vi "SwitchingFieldDistribution.vi"(1 "B":dbl[](array[numeric]), 2 "H":dbl[](array[numeric])) -> (0 "SFD":dbl)   [LabVIEW 2019]
panel:
  out "error out":errorcluster
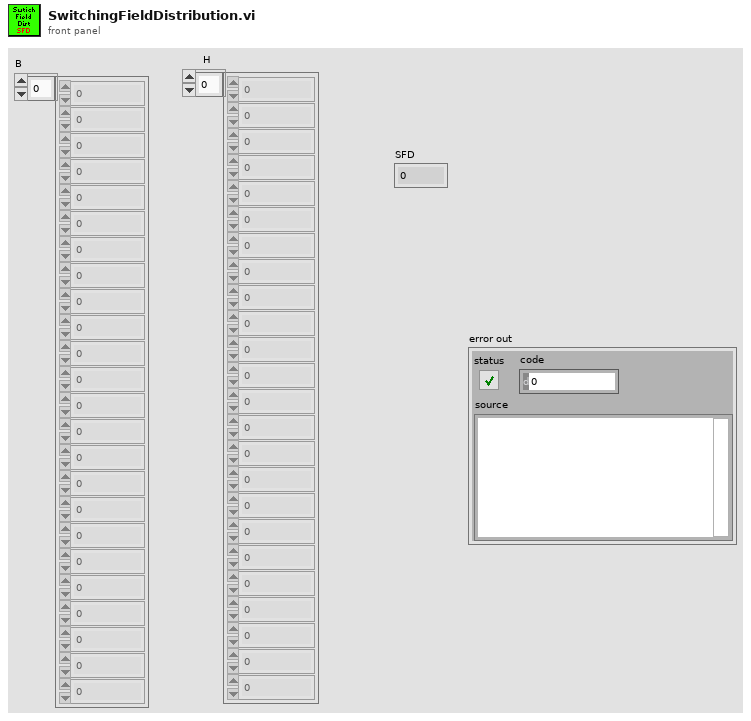
[diagram p1: front panel]
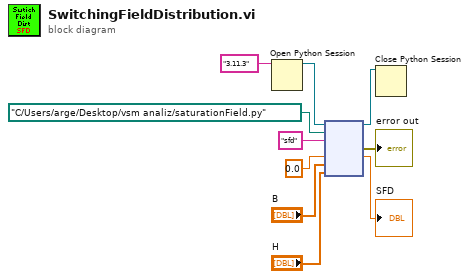
[diagram p0: block diagram]
diagram:
  n1 = Open Python Session(python version="3.11.3" ("Python version")) -> (session out=w6:refnum<k35>)  [unwired: 2 in, 1 out]
  n2 = node(w6, path "C:/Users/arge/Desktop/vsm analiz/saturationField.py" ("module path"), "sfd" ("function name"), 0.0, "B", "H") -> (w5:refnum<k35>, →"error out":errorcluster, →"SFD":dbl)  [unwired: 3 in, 2 out]
  n3 = Close Python Session(session in=w5) -> ()  [unwired: 1 in, 1 out]
